vi "String Trimming 2D to 1D.vi"(7 "Trimming Option":T1=enum."Trimg Empty and Sapce String" caption="Enum 3", 10 "1D String In":string[][](array[string])) -> (2 "1D String Out":string[](array[string]))   [LabVIEW 2024]
uses:
  Typdef/String Trmming Option.ctl
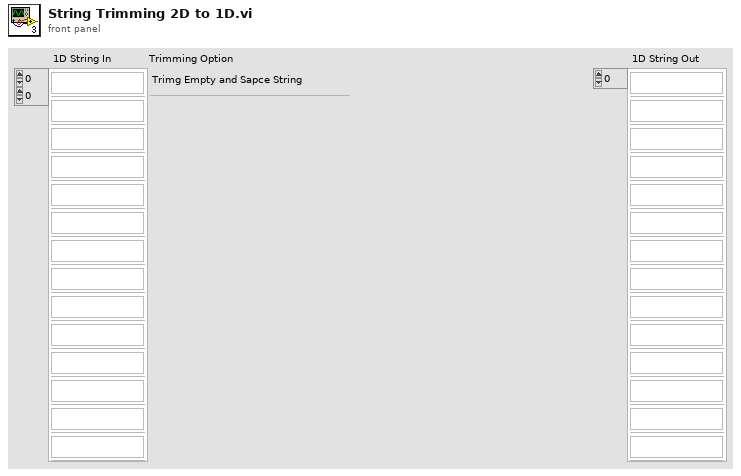
[diagram p1: front panel]
types:
  T1 = typedef "String Trmming Option.ctl" = enum16{"None", "Trim Empty String", "Trim Space String", "Trimg Empty and Sapce String"}
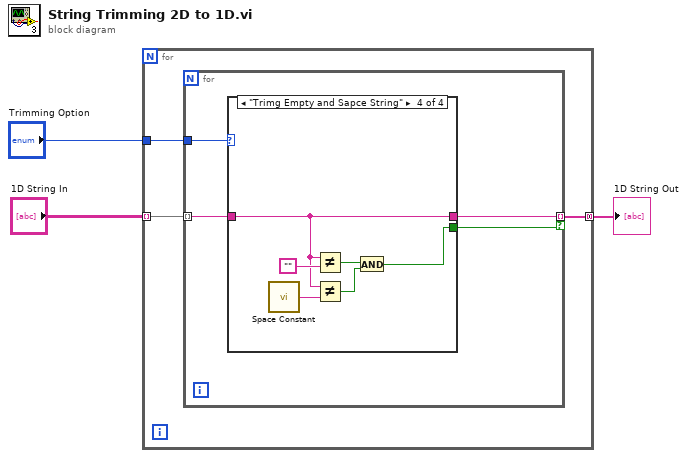
[diagram p0: block diagram]
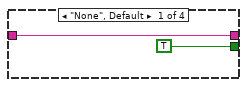
[diagram p2: hidden frame]
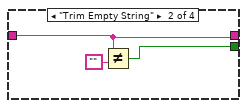
[diagram p3: hidden frame]
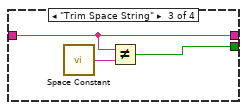
[diagram p4: hidden frame]
diagram:
  n1 = for {
    tunnel: "1D String In" -> [w6] mode=indexing
    tunnel: "Trimming Option" -> [w5]
    tunnel: [w4] -> w1 mode=concatenating
    n2 = for {
      tunnel: w6 -> [w9] mode=indexing
      tunnel: w5 -> [w10]
      tunnel: [w8] -> w4 mode=indexing if=w7
      n3 = case shown="\"Trimg Empty and Sapce String\"" w10 {
        tunnel: w9 -> [w12 w13 w17 w22]
        tunnel: [w12 w13 w17 w22] -> w8
        tunnel: [TRUE w14 w18 w19] -> w7
        frame "None", Default {
        }
        frame "Trim Empty String" {
          n4 = Not Equal?(x=w13, y="") -> (x != y?=w14:bool)
        }
        frame "Trim Space String" {
          n5 = call <vilib>:"Space Constant.vi"() -> ("String"=w16:string)
          n6 = Not Equal?(x=w17, y=w16) -> (x != y?=w18:bool)
        }
        frame "Trimg Empty and Sapce String" {
          n7 = call <vilib>:"Space Constant.vi"() -> ("String"=w23:string)
          n8 = Not Equal?(x=w22, y="") -> (x != y?=w21:bool)
          n9 = Not Equal?(x=w22, y=w23) -> (x != y?=w20:bool)
          n10 = And(x=w21, y=w20) -> (x .and. y?=w19:bool)
        }
      }
    }
  }
  "1D String Out" <- w1
